vi "Dual_image_capture-Talbot.vi"() -> ()   [LabVIEW 2013]
uses:
  <vilib>/DAQmx/create/channels.llb/DAQmx Create Channel (CO-Pulse Generation-Frequency).vi
  <vilib>/DAQmx/configure/timing.llb/DAQmx Timing (Implicit).vi
  <vilib>/vision/driver/NI_Vision_Acquisition_Software.lvlib
  <resource>/objmgr/imaqdx.rc
  <resource>/objmgr/daqmx.rc
panel:
  in  "CO.Pulse.Term":tag="/Dev1/PFI0"
  out "Snap Counter":u32
  in  "Snap":bool
  out "Img #":string
  in  "Gain 2":dbl(slide)=575.0 min=350.0 max=1000.0 step=1.0 scale=350.0..1000.0
  in  "VR2":dbl(slide)=65.0 min=0.0 max=255.0 step=1.0 scale=0.0..255.0
  in  "VR1":dbl(slide)=60.0 min=0.0 max=255.0 step=1.0 scale=0.0..255.0
  in  "UB2":dbl(slide)=160.0 min=0.0 max=255.0 step=1.0 scale=0.0..255.0
  in  "UB1":dbl(slide)=165.0 min=0.0 max=255.0 step=1.0 scale=0.0..255.0
  in  "Shutter":dbl(slide)=4095.0 min=0.0 max=4095.0 step=1.0 scale=4.095..4095.0 scale format="%#.0f"
  in  "Brightness":dbl(slide)=100.0 min=0.0 max=255.0 step=1.0 scale=0.0..255.0
  in  "Gain":dbl(slide)=600.0 min=350.0 max=1000.0 step=1.0 scale=350.0..1000.0
  in  "Test Name":string="test"
  in  "Storage Directory":path=path "C:/Users/Lab_User/Desktop/Users 2011-2012/Michael Rossol"
  out "Image 2":T1(plugin-control)
  out "Buffer Number 2":u32
  out "Frame Rate 2":dbl
  in  "Camera Name 2":refnum<k21>="cam1" caption="IMAQdx Session"
  in  "Images per \nsecond (hz)":dbl=2.0 format="%.1f"
  out "Actual Duty Cycle":dbl
  out "Actual Frequency":dbl
  in  "Stop":bool
  in  "Start Trigger Mode":bool
  out "Frame Rate 1":dbl
  out "Buffer Number 1":u32
  in  "Camera Name 1":refnum<k21>="cam0" caption="IMAQdx Session"
  out "Image":T1(plugin-control)
  # "Exposure Settings - Both Cameras"
  # "White Balance - Camera1"
  # "White Balance - Camera2"
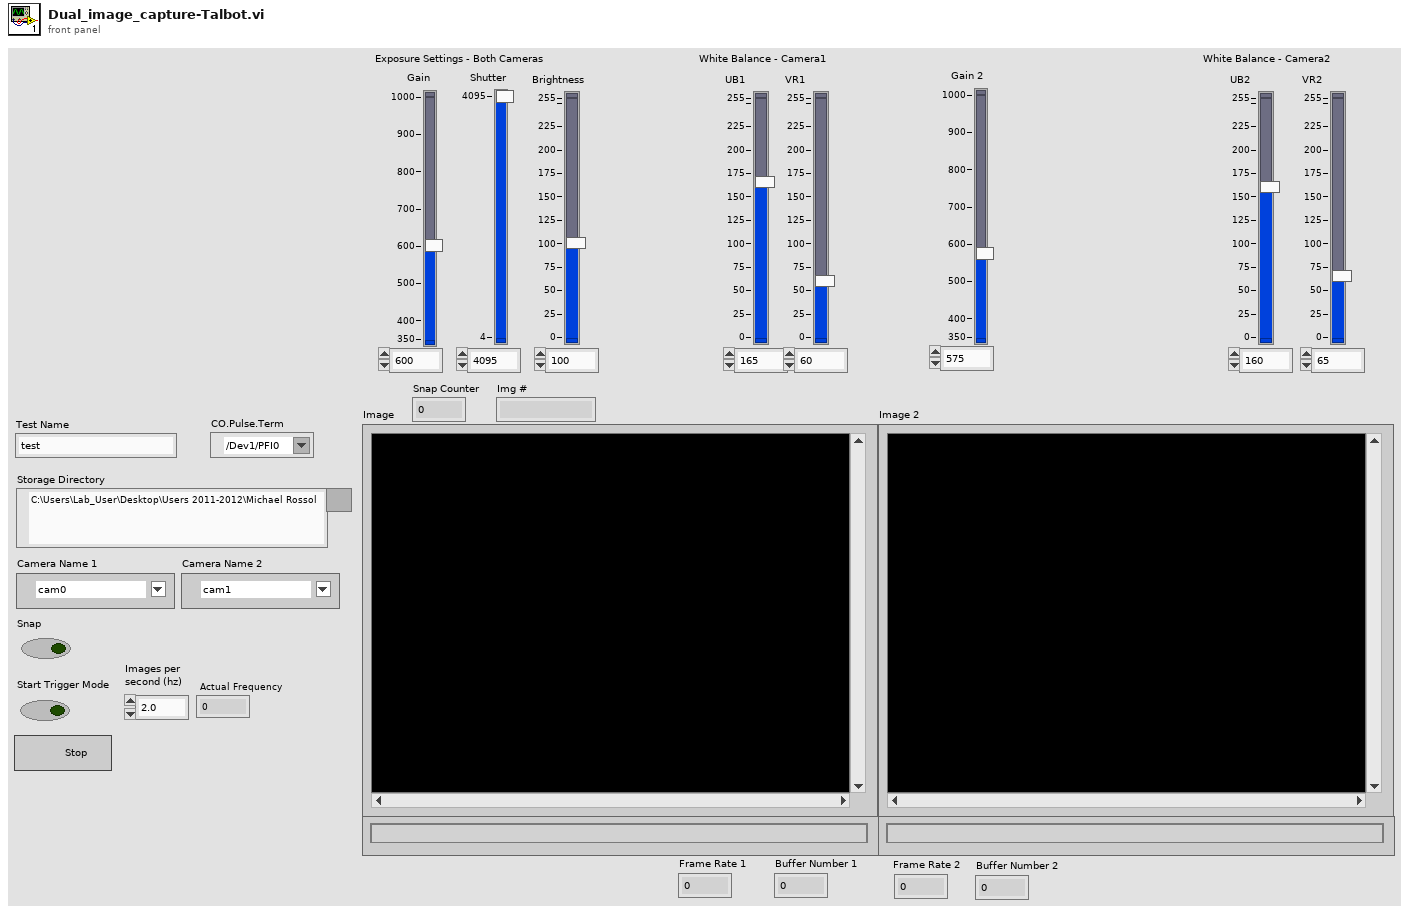
[diagram p1: front panel]
types:
  T1 = typedef "IMAQ Image.ctl" = refnum<image>
  T2 = enum16{"open", "open or create", "create or replace", "create", "open (read only)"}
  T3 = typedef "IMAQdx.ctl" = refnum<k21>
  T4 = enum16{"open", "replace", "create", "open or create", "replace or create", "replace or create with confirmation"}
  T5 = cluster{"Trigger Mode":u32, "Trigger Activation":u32, "Timeout (ms)":u32}
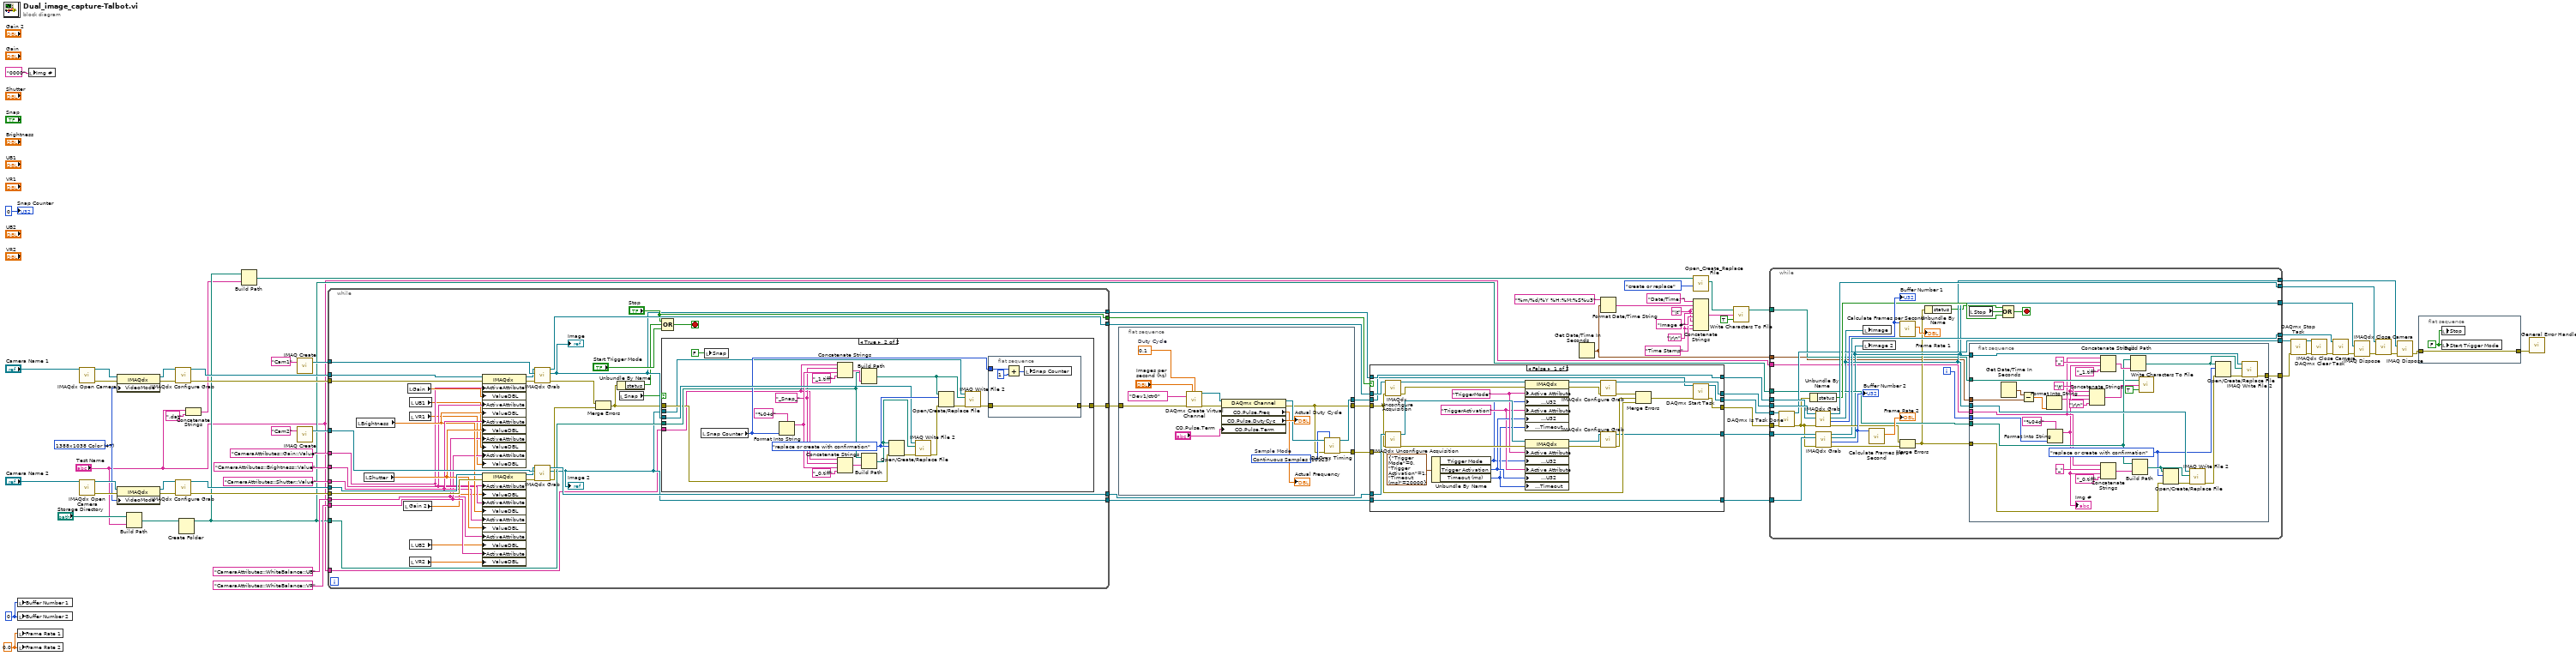
[diagram p0: block diagram]
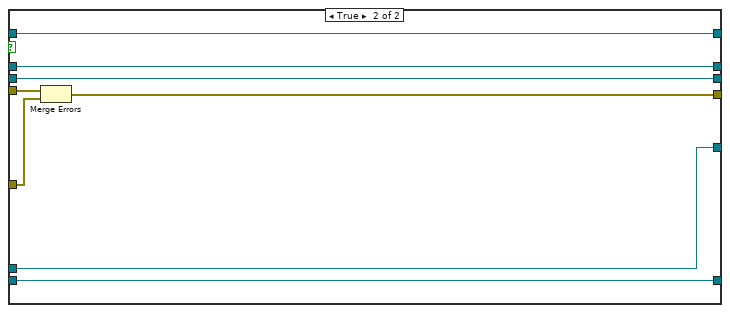
[diagram p2: hidden frame]
diagram:
  w6 = "\t"
  w9 = "\r\n"
  w35 = u32 47 items=["320x240 Color"=4, "640x480 Mono8"=9, "640x480 Mono16"=19, "640x480 Color"=14, "800x600 Mono8"=21, "800x600 Mono16"=27, "800x600 Color"=24, "1024x768 Mono8"=30, "1024x768 Mono16"=36, "1024x768 Color"=33, "1280x960 Mono8"=40, "1280x960 Mono16"=46, "1280x960 Color"=43, "1388x1038 Color"=47, "1388x1038 Mono"=48] ("Video Mode")
  w36 = 0.0 ("Frame Rate 1")
  w37 = u32 0 ("Buffer Number 1")
  n1 = local write "Buffer Number 1"(w37) -> ()
  n2 = local write "Buffer Number 2"(w37) -> ()
  n3 = local write "Frame Rate 1"(w36) -> ()
  n4 = local write "Frame Rate 2"(w36) -> ()
  n5 = local write "Img #"("0000" ("im num 2")) -> ()
  n6 = call <vilib>:"IMAQdx Open Camera.vi"("Session In"="Camera Name 1") -> ("error out"=w43:errorcluster, "Session Out"=w45:T3)  [unwired: 2 in, 7 out]
  n7 = call <vilib>:"IMAQdx Open Camera.vi"("Session In"="Camera Name 2") -> ("error out"=w38:errorcluster, "Session Out"=w39:T3)  [unwired: 2 in, 7 out]
  n8 = property class="IMAQdx"(reference=w45, error in=w43, "VideoMode"=w35) -> (reference out=w44:T3, error out=w42:errorcluster)
  n9 = property class="IMAQdx"(reference=w39, error in=w38, "VideoMode"=w35) -> (reference out=w41:T3, error out=w40:errorcluster)
  n10 = Build Path(base path="Storage Directory", name or relative path="Test Name") -> (appended path=w4:path)
  n11 = call <vilib>:"IMAQdx Configure Grab.vi"("error in"=w42, "Session In"=w44) -> ("error out"=w66:errorcluster, "Session Out"=w67:T3)  [unwired: 8 out]
  n12 = call <vilib>:"IMAQdx Configure Grab.vi"("error in"=w40, "Session In"=w41) -> ("error out"=w57:errorcluster, "Session Out"=w58:T3)  [unwired: 8 out]
  n13 = Create Folder(path (use dialog)=w4) -> (created path=w12:path)  [unwired: 2 in, 2 out]
  n14 = Concatenate Strings("Test Name", ".dat" ("string")) -> (w2:string)
  n15 = Build Path(base path=w12, name or relative path=w2) -> (appended path=w20:path)
  n16 = call "IMAQ Create"("Image Name"="Cam1") -> ("New Image"=w68:T1)  [unwired: 3 in, 2 out]
  n17 = call "IMAQ Create"("Image Name"="Cam2") -> ("New Image"=w32:T1)  [unwired: 3 in, 2 out]
  n18 = while {
    tunnel: [w115] -> w75
    tunnel: w66 -> [w108]
    tunnel: w67 -> [w110]
    tunnel: w68 -> [w112]
    tunnel: [w84] -> w63
    tunnel: ["Stop"] -> w64
    tunnel: w58 -> [w106]
    tunnel: w57 -> [w105]
    tunnel: [w85] -> w34
    tunnel: [w113] -> w56
    tunnel: [w80] -> w55
    tunnel: w32 -> [w111]
    tunnel: "CameraAttributes::Shutter::Value" ("ActiveAttribute") -> [w101]
    tunnel: "CameraAttributes::Brightness::Value" ("ActiveAttribute") -> [w99]
    tunnel: "CameraAttributes::Gain::Value" ("ActiveAttribute") -> [w97]
    tunnel: "CameraAttributes::WhiteBalance::UB" ("ActiveAttribute") -> [w94]
    tunnel: "CameraAttributes::WhiteBalance::VR" ("ActiveAttribute") -> [w95]
    tunnel: w12 -> [w82]
    tunnel: "Test Name" -> [w78]
    stop <- w89 stop-if-true
    n19 = local read "Brightness"() -> (w100:dbl)
    n20 = local read "Shutter"() -> (w102:dbl)
    n21 = local read "Gain 2"() -> (w90:dbl)
    n22 = local read "Gain"() -> (w98:dbl)
    n23 = local read "UB1"() -> (w96:dbl)
    n24 = local read "VR1"() -> (w92:dbl)
    n25 = local read "UB2"() -> (w93:dbl)
    n26 = local read "VR2"() -> (w91:dbl)
    n27 = property class="IMAQdx"(reference=w110, error in=w108, "ActiveAttribute"=w97, "ValueDBL"=w98, "ActiveAttribute"=w99, "ValueDBL"=w100, "ActiveAttribute"=w101, "ValueDBL"=w102, "ActiveAttribute"=w94, "ValueDBL"=w96, "ActiveAttribute"=w95, "ValueDBL"=w92) -> (reference out=w109:T3, error out=w107:errorcluster)
    n28 = property class="IMAQdx"(reference=w106, error in=w105, "ActiveAttribute"=w97, "ValueDBL"=w90, "ActiveAttribute"=w99, "ValueDBL"=w100, "ActiveAttribute"=w101, "ValueDBL"=w102, "ActiveAttribute"=w94, "ValueDBL"=w93, "ActiveAttribute"=w95, "ValueDBL"=w91) -> (reference out=w103:T3, error out=w104:errorcluster)
    n29 = call <vilib>:"IMAQdx Grab.vi"("error in"=w107, "Image In"=w112, "Session In"=w109) -> ("error out"=w88:errorcluster, "Image Out"=w84:T1, "Session Out"=w115:T3)  [unwired: 1 in, 5 out]
    "Image" <- w84
    n30 = call <vilib>:"IMAQdx Grab.vi"("error in"=w104, "Image In"=w111, "Session In"=w103) -> ("error out"=w86:errorcluster, "Image Out"=w80:T1, "Session Out"=w113:T3)  [unwired: 1 in, 5 out]
    "Image 2" <- w80
    n31 = Merge Errors(w88, w86) -> (w83:errorcluster)
    n32 = Unbundle By Name(w83) -> ("status"=w79:bool)
    n33 = local read "Snap"() -> (w81:bool)
    n34 = Compound Arithmetic op=OR("Stop", w79, "Start Trigger Mode") -> (w89:bool)
    n35 = case shown="True" w81 {
      tunnel: [w116 w123] -> w85
      tunnel: w84 -> [_ w127]
      tunnel: w82 -> [_ w121]
      tunnel: w83 -> [w116 w120]
      tunnel: w80 -> [_ w119]
      tunnel: w78 -> [_ w117]
      frame False {
      }
      frame True {
        w118 = "_Snap_"
        w130 = T4."replace or create with confirmation" ("operation (0:open)")
        n36 = local read "Snap Counter"() -> (w125:u32)
        n37 = local write "Snap"(FALSE ("Ready?")) -> ()
        n38 = Format Into String(format string="%04d", w125) -> (resulting string=w122:string)  [unwired: 2 in, 1 out]
        n39 = Concatenate Strings(w117, w118, w122, "_1.tiff") -> (w134:string)
        n40 = Concatenate Strings(w117, w118, w122, "_0.tiff") -> (w135:string)
        n41 = Build Path(base path=w121, name or relative path=w134) -> (appended path=w129:path)
        n42 = Build Path(base path=w121, name or relative path=w135) -> (appended path=w128:path)
        n43 = Open/Create/Replace File(file path (use dialog)=w128, error in=w120, operation (0:open)=w130) -> (error out=w131:errorcluster)  [unwired: 3 in, 2 out]
        n44 = call-poly "IMAQ Write File 2"("error in (no error)"=w131, "File Path"=w128, "Image"=w127) -> ("error out"=w133:errorcluster)  [unwired: 7 in, 1 out]
        n45 = Open/Create/Replace File(file path (use dialog)=w129, error in=w133, operation (0:open)=w130) -> (error out=w132:errorcluster)  [unwired: 3 in, 2 out]
        n46 = call-poly "IMAQ Write File 2"("error in (no error)"=w132, "File Path"=w129, "Image"=w119) -> ("error out"=w124:errorcluster)  [unwired: 7 in, 1 out]
        n47 = flat-sequence {
          tunnel: w125 -> [w142]
          tunnel: w124 -> [w139]
          tunnel: [w139] -> w123
          frame #0 {
            n48 = Add(x=w142, y=u32 1) -> (x+y=w140:u32)
            n49 = local write "Snap Counter"(w140) -> ()
          }
        }
      }
    }
  }
  n50 = flat-sequence {
    tunnel: [w147] -> w61
    tunnel: [w146] -> w54
    tunnel: w34 -> [w145]
    tunnel: [w144] -> w33
    frame #0 {
      w154 = 0.1  # Duty Cycle
      w148 = 10123 items=["Finite Samples"=10178, "Continuous Samples"=10123, "Hardware Timed Single Point"=12522]  # Sample Mode
      n51 = call-poly <vilib>:"DAQmx Create Virtual Channel.vi"("frequency"="Images per \nsecond (hz)", "duty cycle"=w154, "counter"=tag "Dev1/ctr0" ("Counter"), "error in"=w145) -> ("task out"=w150:refnum<k21>, "error out"=w151:errorcluster)  [unwired: 10 in]
      n52 = property class="DAQmx Channel"(reference=w150, error in=w151, "CO.Pulse.Term"="CO.Pulse.Term") -> (reference out=w152:refnum<k21>, error out=w144:errorcluster, "CO.Pulse.Freq"=→"Actual Frequency":dbl, "CO.Pulse.DutyCyc"=→"Actual Duty Cycle":dbl)
      n53 = call-poly <vilib>:"DAQmx Timing.vi"("task/channels in"=w152, "sample mode"=w148, "error in"=w144) -> ("task out"=w147:refnum<k21>, "error out"=w146:errorcluster)  [unwired: 11 in]
    }
  }
  n54 = case shown="False" w64 {
    tunnel: w75 -> [w184 w192]
    tunnel: [w183 w192] -> w74
    tunnel: [w165 w185] -> w11
    tunnel: [w166 w190] -> w72
    tunnel: w63 -> [w177 w191]
    tunnel: [w177 w191] -> w62
    tunnel: w61 -> [w158 w190]
    tunnel: w33 -> [w157 w189]
    tunnel: w56 -> [w168 w186]
    tunnel: w55 -> [w167 w187]
    tunnel: [w167 w187] -> w53
    tunnel: w54 -> [w161 w188]
    tunnel: [w159 w186] -> w52
    frame False {
      w171 = "TriggerActivation" ("ActiveAttribute")
      w173 = "TriggerMode" ("ActiveAttribute")
      n55 = call <vilib>:"IMAQdx Unconfigure Acquisition.vi"("error in"=w157, "Session In"=w184) -> ("error out"=w180:errorcluster, "Session Out"=w179:T3)  [unwired: 8 out]
      n56 = call <vilib>:"IMAQdx Unconfigure Acquisition.vi"("error in"=w157, "Session In"=w168) -> ("error out"=w175:errorcluster, "Session Out"=w174:T3)  [unwired: 8 out]
      n57 = Unbundle By Name(T5 {"Trigger Mode"=0, "Trigger Activation"=1, "Timeout (ms)"=20000} ("Trigger Parameters")) -> ("Trigger Mode"=w169:u32, "Trigger Activation"=w172:u32, "Timeout (ms)"=w170:u32)
      n58 = property class="IMAQdx"(reference=w179, error in=w180, "Camera Attributes:Active Attribute"=w173, "Camera Attributes:Value:U32"=w169, "Camera Attributes:Active Attribute"=w171, "Camera Attributes:Value:U32"=w172, "Acquisition Attributes:Timeout"=w170) -> (reference out=w181:T3, error out=w182:errorcluster)
      n59 = property class="IMAQdx"(reference=w174, error in=w175, "Camera Attributes:Active Attribute"=w173, "Camera Attributes:Value:U32"=w169, "Camera Attributes:Active Attribute"=w171, "Camera Attributes:Value:U32"=w172, "Acquisition Attributes:Timeout"=w170) -> (reference out=w176:T3, error out=w164:errorcluster)
      n60 = call <vilib>:"IMAQdx Configure Grab.vi"("error in"=w182, "Session In"=w181) -> ("error out"=w160:errorcluster, "Session Out"=w183:T3)  [unwired: 8 out]
      n61 = call <vilib>:"IMAQdx Configure Grab.vi"("error in"=w164, "Session In"=w176) -> ("error out"=w162:errorcluster, "Session Out"=w159:T3)  [unwired: 8 out]
      n62 = Merge Errors(w160, w162, w161) -> (w163:errorcluster)
      n63 = call <vilib>:"DAQmx Start Task.vi"("task/channels in"=w158, "error in"=w163) -> ("task out"=w166:refnum<k21>, "error out"=w165:errorcluster)  [unwired: 12 in]
    }
    frame True {
      n64 = Merge Errors(w189, w188) -> (w185:errorcluster)
    }
  }
  n65 = Get Date/Time In Seconds() -> (seconds since 1Jan1904=w3:timestamp)
  n66 = Format Date/Time String(time format string (%c)="%m/%d/%Y %H:%M:%S%u3", seconds (now)=w3) -> (date/time string=w7:string)  [unwired: 1 in]
  n67 = call <vilib>:"Open_Create_Replace File.vi"("function (open:0)"=T2."create or replace", "file path"=w20) -> ("new file path"=w24:path)  [unwired: 6 in, 3 out]
  n68 = Concatenate Strings("Date/Time: ", w7, w6, w9, "Image #", w6, "Time Stamp" ("string"), w9) -> (w22:string)
  n69 = call <vilib>:"Write Characters To File.vi"("append to file? (new file:F)"=TRUE, "character string"=w22, "file path (dialog if empty)"=w24) -> ("new file path (Not A Path if cancelled)"=w5:path)  [unwired: 2 in]
  n70 = while {
    tunnel: [w221] -> w70
    tunnel: [w199] -> w17
    tunnel: w74 -> [w218]
    tunnel: w62 -> [w217]
    tunnel: [w214] -> w69
    tunnel: w72 -> [w213]
    tunnel: w53 -> [w210]
    tunnel: w52 -> [w209]
    tunnel: w11 -> [w206]
    tunnel: [w203] -> w46
    tunnel: [w202] -> w48
    tunnel: [w205] -> w47
    tunnel: w12 -> [w204]
    tunnel: w5 -> [w196]
    tunnel: "Test Name" -> [w194]
    tunnel: w3 -> [w193]
    i -> [w197]
    stop <- w215 stop-if-true
    n71 = call <vilib>:"DAQmx Is Task Done.vi"("task/channels in"=w213, "error in"=w206) -> ("task out"=w214:refnum<k21>, "error out"=w200:errorcluster)  [unwired: 11 in, 1 out]
    n72 = Unbundle By Name(w200) -> ("status"=w216:bool)
    n73 = call <vilib>:"IMAQdx Grab.vi"("error in"=w200, "Image In"=w217, "Session In"=w218) -> ("error out"=w207:errorcluster, "Buffer Number Out"=w219:u32, "Image Out"=w203:T1, "Session Out"=w221:T3)  [unwired: 1 in, 4 out]
    "Buffer Number 1" <- w219
    n74 = call <vilib>:"IMAQdx Grab.vi"("error in"=w200, "Image In"=w210, "Session In"=w209) -> ("error out"=w201:errorcluster, "Buffer Number Out"=w208:u32, "Image Out"=w202:T1, "Session Out"=w205:T3)  [unwired: 1 in, 4 out]
    "Buffer Number 2" <- w208
    n75 = local write "Image"(w203) -> ()
    n76 = local write "Image 2"(w202) -> ()
    n77 = call <vilib>:"Calculate Frames per Second.vi"("Buffer Number"=w208) -> ("Processed Frames/s"=→"Frame Rate 2":dbl)  [unwired: 8 in, 2 out]
    n78 = call <vilib>:"Calculate Frames per Second.vi"("Buffer Number"=w219) -> ("Processed Frames/s"=→"Frame Rate 1":dbl)  [unwired: 8 in, 2 out]
    n79 = Merge Errors(w207, w201) -> (w198:errorcluster)
    n80 = Unbundle By Name(w198) -> ("status"=w195:bool)
    n81 = local read "Stop"() -> (w212:bool)
    n82 = flat-sequence {
      tunnel: w204 -> [w235]
      tunnel: w203 -> [w251]
      tunnel: w202 -> [w250]
      tunnel: w198 -> [w249]
      tunnel: [w248] -> w199
      tunnel: w197 -> [w239]
      tunnel: w196 -> [w233]
      tunnel: w194 -> [w227]
      tunnel: w193 -> [w224]
      frame #0 {
        w245 = T4."replace or create with confirmation" ("operation (0:open)")
        n83 = Get Date/Time In Seconds() -> (seconds since 1Jan1904=w225:timestamp)
        n84 = Subtract(x=w225, y=w224) -> (x-y=w223:dbl)
        n85 = Format Into String(w223) -> (resulting string=w222:string)  [unwired: 3 in, 1 out]
        n86 = Format Into String(format string="%04d", w239) -> (resulting string=w226:string)  [unwired: 2 in, 1 out]
        "Img #" <- w226
        n87 = Concatenate Strings(w226, "\t", w222, "\r\n") -> (w232:string)
        n88 = Concatenate Strings(w227, "_" ("string"), w226, "_1.tiff") -> (w241:string)
        n89 = Concatenate Strings(w227, "_" ("string"), w226, "_0.tiff") -> (w240:string)
        n90 = Build Path(base path=w235, name or relative path=w241) -> (appended path=w246:path)
        n91 = Build Path(base path=w235, name or relative path=w240) -> (appended path=w247:path)
        n92 = call <vilib>:"Write Characters To File.vi"("append to file? (new file:F)"=TRUE, "character string"=w232, "file path (dialog if empty)"=w233) -> ()  [unwired: 2 in, 1 out]
        n93 = Open/Create/Replace File(file path (use dialog)=w247, error in=w249, operation (0:open)=w245) -> (error out=w244:errorcluster)  [unwired: 3 in, 2 out]
        n94 = call-poly "IMAQ Write File 2"("error in (no error)"=w244, "File Path"=w247, "Image"=w251) -> ("error out"=w242:errorcluster)  [unwired: 7 in, 1 out]
        n95 = Open/Create/Replace File(file path (use dialog)=w246, error in=w242, operation (0:open)=w245) -> (error out=w243:errorcluster)  [unwired: 3 in, 2 out]
        n96 = call-poly "IMAQ Write File 2"("error in (no error)"=w243, "File Path"=w246, "Image"=w250) -> ("error out"=w248:errorcluster)  [unwired: 7 in, 1 out]
      }
    }
    n97 = Compound Arithmetic op=OR(w195, w212, w216) -> (w215:bool)
  }
  n98 = call <vilib>:"DAQmx Stop Task.vi"("task/channels in"=w69, "error in"=w17) -> ("task out"=w71:refnum<k21>, "error out"=w73:errorcluster)  [unwired: 12 in]
  n99 = call <vilib>:"DAQmx Clear Task.vi"("task in"=w71, "error in"=w73) -> ("error out"=w49:errorcluster)  [unwired: 13 in]
  n100 = call <vilib>:"IMAQdx Close Camera.vi"("error in"=w49, "Session In"=w47) -> ("error out"=w51:errorcluster)  [unwired: 9 out]
  n101 = call "IMAQ Dispose"("Image"=w48, "error in (no error)"=w51) -> ("error out"=w50:errorcluster)  [unwired: 4 in]
  n102 = call <vilib>:"IMAQdx Close Camera.vi"("error in"=w50, "Session In"=w70) -> ("error out"=w77:errorcluster)  [unwired: 9 out]
  n103 = call "IMAQ Dispose"("Image"=w46, "error in (no error)"=w77) -> ("error out"=w14:errorcluster)  [unwired: 4 in]
  n104 = flat-sequence {
    tunnel: w14 -> [w252]
    tunnel: [w252] -> w16
    frame #0 {
      w253 = FALSE ("Stop")
      n105 = local write "Stop"(w253) -> ()
      n106 = local write "Start Trigger Mode"(w253) -> ()
    }
  }
  n107 = call <vilib>:"General Error Handler.vi"("error in (no error)"=w16) -> ()  [unwired: 1 in, 14 out]
  "Snap Counter" <- u32 0 ("Snap Counter")
